vi "Elevator Immediate.vi"(6 "Synchronication":enum16{"Start", "Wait"}(ring), 7 "Description":string, 8 "Command Info In":T2, 10 "Position":T1, 11 "Setpoint":dbl) -> (0 "Command Info Out":T2)   [LabVIEW 2018]
doc: "This template is useful for immediate subsystem actions that do not need deadband filtering\n\nBe sure to right-click and select New from Template and save with a new command name."
uses:
  <vilib>/Rock Robotics/WPI/Framework/Command Status Info.ctl
  <vilib>/Rock Robotics/WPI/Framework/Completion Status.ctl
  <vilib>/Rock Robotics/WPI/Framework/Completion Notifier.ctl
  Implementation/Infrastructure/Positions.ctl
  Implementation/Elevator Operations.ctl
  Implementation/Elevator Setpoints.ctl
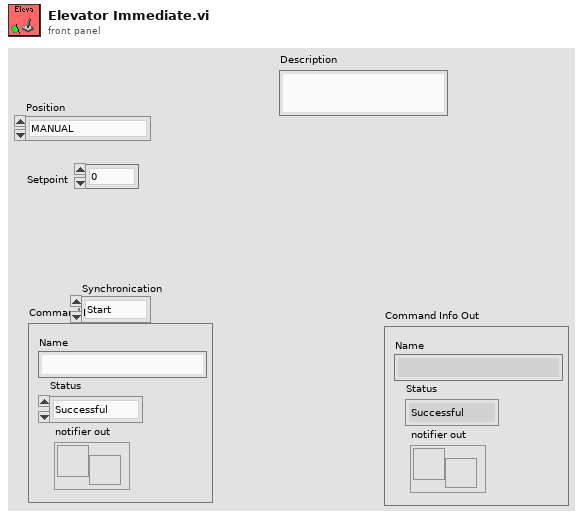
[diagram p1: front panel]
types:
  T1 = typedef "Positions.ctl" = enum16{"MANUAL", "Bottom Pannel", "Bottom Cargo", "Feeder Station", "Cargo Ship Cargo", "Middle Pannel", "Middle Cargo", "Top Pannel", "Top Cargo"}
  T2 = typedef "Command Status Info.ctl" = cluster{"Name":string, "Status":T3, "notifier out":T4}
  T3 = typedef "Completion Status.ctl" = enum16{"Successful", "Aborted", "Incomplete"}
  T4 = typedef "Completion Notifier.ctl" = refnum<notifier>
  T5 = typedef "Elevator Operations.ctl" = enum16{"Reserve", "Read Current", "Immediate"}
  T6 = typedef "Elevator Setpoints.ctl" = cluster{"Operation":T5, "Manual Input":dbl, "Position":T1, "1/3 Power":bool}
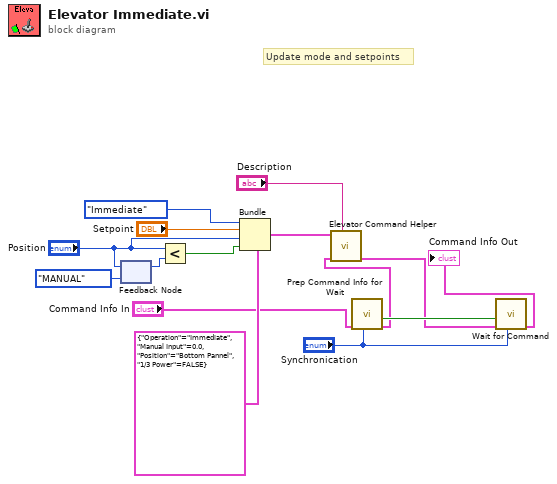
[diagram p0: block diagram]
diagram:
  # "Update mode and setpoints"
  n1 = feedback-in #1("Position") -> ()
  n2 = feedback #1(Positions."MANUAL" ("Position")) -> (w10:T1)
  n3 = Less?(x="Position", y=w10) -> (x < y?=w7:bool)
  n4 = Bundle(cluster=T6 {"Operation"=enum."Immediate", "Manual Input"=0.0, "Position"=enum."Bottom Pannel", "1/3 Power"=FALSE} ("SubSystem Data"), "Operation"=Elevator_Operations."Immediate", "Manual Input"="Setpoint", "Position"="Position", "1/3 Power"=w7) -> (w13:T6)
  n5 = call <vilib>:"Prep Command Info for Wait.vi"("Synchronication"="Synchronication", "Command Info"="Command Info In") -> ("Command Info"=w3:T2, "Allocated"=w6:bool)  [unwired: 8 in]
  n6 = call "Elevator Command Helper.vi"("Description"="Description", "Command Info In"=w3, "SubSystem Data"=w13) -> ("Command Info Out"=w2:T2)  [unwired: 6 in, 2 out]
  n7 = call <vilib>:"Wait for Command.vi"("Synchronication"="Synchronication", "Command Info in"=w2, "Allocated"=w6) -> ("Command Info out"=→"Command Info Out":T2)  [unwired: 8 in]
